vi "Destroy.vi"(8 "error in (no error)":errorcluster, 11 "XRay Part Sample in":refnum<class "XRay Part Sample.lvclass">) -> (0 "error out":errorcluster, 3 "XRay Part Sample out":refnum<class "XRay Part Sample.lvclass">)   [LabVIEW 2026, in "XRay Part Sample.lvclass"]
uses:
  XRay Part Sample.lvclass
  XRay Part Sample.lvclass/XRay Part Sample.ctl
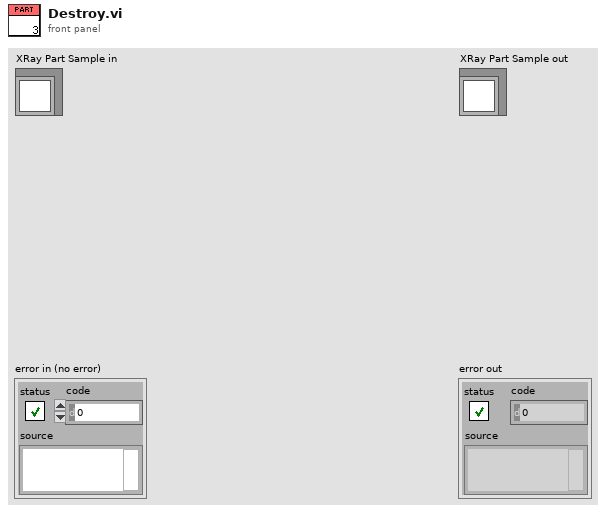
[diagram p1: front panel]
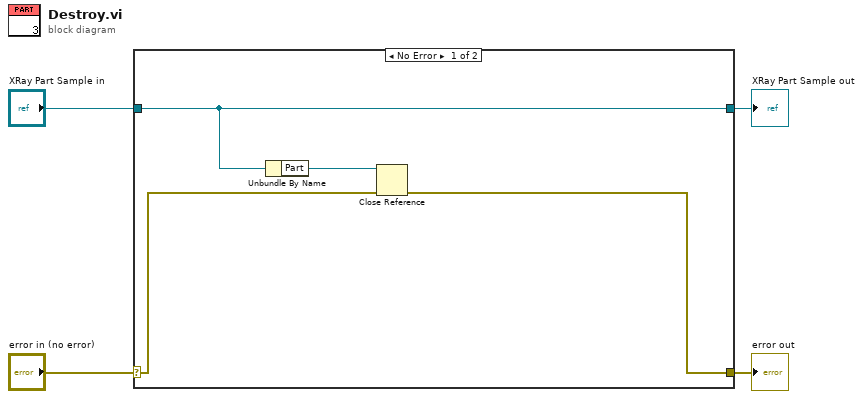
[diagram p0: block diagram]
diagram:
  n1 = case shown="No Error" "error in (no error)" {
    selector: "error in (no error)" -> [w6 w10]
    tunnel: [w5 w10] -> w3
    tunnel: [w8 w9] -> w1
    tunnel: "XRay Part Sample in" -> [w8 w9]
    frame No Error {
      n2 = Unbundle By Name(w8) -> ("Part"=w7:refnum<vi>)
      n3 = Close Reference(reference=w7, error in (no error)=w6) -> (error out=w5:errorcluster)
    }
    frame Error {
    }
  }
  "error out" <- w3
  "XRay Part Sample out" <- w1
